vi "queryPosition.vi"(0 "VISA资源名称":refnum<visa-resource-name>) -> (1 "VISA资源名称 2":refnum<visa-resource-name>, 2 "数值":dbl)   [LabVIEW 2018]
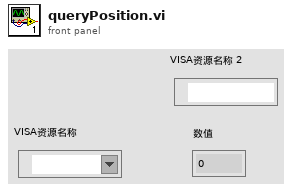
[diagram p1: front panel]
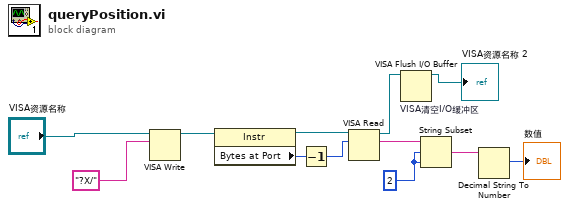
[diagram p0: block diagram]
diagram:
  w2 = 2
  n1 = VISA Write(VISA resource name="VISA资源名称", write buffer="?X/") -> (VISA resource name out=w11:refnum<visa-resource-name>)  [unwired: 1 in, 2 out]
  n2 = property class="Instr"(reference=w11) -> (reference out=w10:refnum<visa-resource-name>, "Bytes at Port"=w8:u32)  [unwired: 1 in, 1 out]
  n3 = Decrement(x=w8) -> (x-1=w7:u32)
  n4 = VISA Read(VISA resource name=w10, byte count=w7) -> (VISA resource name out=w6:refnum<visa-resource-name>, read buffer=w5:string)  [unwired: 1 in, 2 out]
  n5 = VISA Flush I/O Buffer "VISA清空I/O缓冲区"(VISA resource name=w6) -> (VISA resource name out=→"VISA资源名称 2":refnum<visa-resource-name>)  [unwired: 2 in, 1 out]
  n6 = String Subset(string=w5, offset (0)=w2, length (rest)=w2) -> (substring=w4:string)
  n7 = Decimal String To Number(string=w4) -> (number=→"数值":i32)  [unwired: 2 in, 1 out]
